vi "Read Element of Seq_GUI.vi"(8 "error in (no error)":errorcluster, 10 "Variant":T1=enum."Testing", 11 "GUI_Handler_Main in":refnum<class "GUI_Handler_Main.lvclass">) -> (0 "error out":errorcluster, 2 "GUI_Handler_Seq.lvclass":refnum<class "GUI_Handler_Seq.lvclass">, 3 "GUI_Handler_Main out":refnum<class "GUI_Handler_Main.lvclass">)   [LabVIEW 2017, in "GUI_Handler_Main.lvclass"]
uses:
  GUI_Handler_Main.lvclass
  GUIHandler/GUI_Handler_Seq.lvclass
  Typedef/TestTypeSelect.ctl
  GUIHandler/GuiSectionEnum.ctl
  GUI_Handler_Main.lvclass/GUI_Handler_Main.ctl
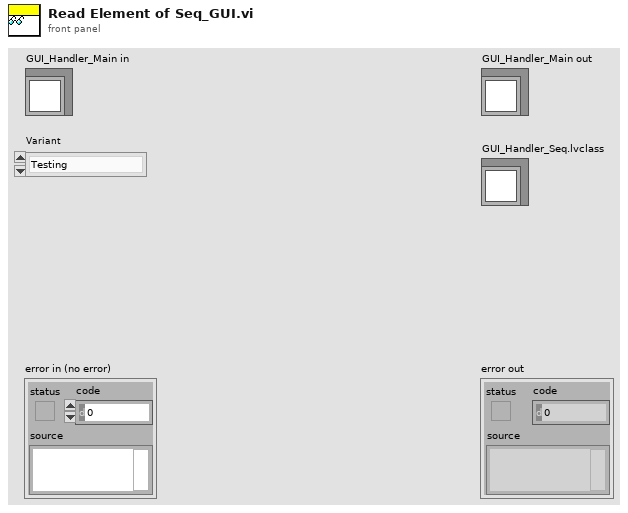
[diagram p1: front panel]
types:
  T1 = typedef "TestTypeSelect.ctl" = enum16{"Calibration", "Testing"}
  T2 = typedef "GuiSectionEnum.ctl" = enum16{"TestingSection", "CalibrationSection"}
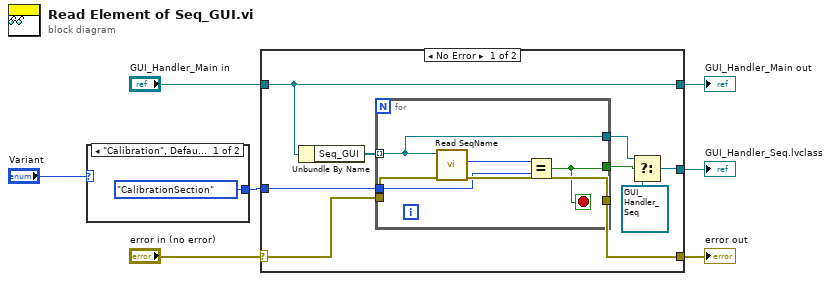
[diagram p0: block diagram]
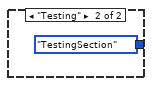
[diagram p2: hidden frame]
diagram:
  n1 = case shown="\"Calibration\", Default" "Variant" {
    tunnel: [GuiSectionEnum."CalibrationSection" ("y") GuiSectionEnum."TestingSection" ("y")] -> w1
    frame "Calibration", Default {
    }
    frame "Testing" {
    }
  }
  n2 = case shown="No Error" "error in (no error)" {
    selector: "error in (no error)" -> [w16 w25]
    tunnel: [w15 w25] -> w6
    tunnel: [w18 w26] -> w4
    tunnel: "GUI_Handler_Main in" -> [w18 w26]
    tunnel: [w14 _] -> w3
    tunnel: w1 -> [w10 _]
    frame No Error {
      n3 = Unbundle By Name(w18) -> ("Seq_GUI"=w17:refnum<class "GUI_Handler_Seq.lvclass">[])
      n4 = for {
        tunnel: w17 -> [w22] mode=indexing
        tunnel: w16 -> [w24]
        tunnel: [w23] -> w15
        tunnel: [w22] -> w12
        tunnel: [w21] -> w13
        tunnel: w10 -> [w19]
        stop <- w21 stop-if-true
        n5 = call-dynamic "Read SeqName.vi"("error in (no error)"=w24, "GUI_Handler_Seq in"=w22) -> ("error out"=w23:errorcluster, "SeqName"=w20:T2)  [unwired: 7 in, 1 out]
        n6 = Equal?(x=w20, y=w19) -> (x = y?=w21:bool)
      }
      n7 = Select(t=w12, s=w13, f=refnum<class "GUI_Handler_Seq.lvclass"> refnum) -> (s? t:f=w14:refnum<class "GUI_Handler_Seq.lvclass">)
    }
    frame Error {
    }
  }
  "error out" <- w6
  "GUI_Handler_Main out" <- w4
  "GUI_Handler_Seq.lvclass" <- w3
